vi "Obtain Control Cluster.vi"(9 "I/O":bool=TRUE, 10 "Dispense":bool=TRUE, 11 "Motion":bool=TRUE) -> (3 "Control Out":T1)   [LabVIEW 2020, in "Controller.lvclass"]
uses:
  Controller.lvclass
  Controllers.ctl
  I-O/I-O.lvclass
  Dispenser/Dispenser.lvclass
  C:/Program Files (x86)/Aerotech/A3200/LabVIEW/2010/Bin/Aerotech.A3200.dll
  Program Files (x86)/Aerotech/A3200/LabVIEW/2010/Bin/Aerotech.A3200.dll
  I-O/NI-DAQ/NI-DAQ.lvclass
  C:/Users/hep/Documents/CMU gantry/Classes/Controller/I-O/I-O.lvclass
  Dispenser/Ultimus V/Ultimus V.lvclass
  C:/Users/hep/Documents/CMU gantry/Classes/Controller/Dispenser/Dispenser.lvclass
panel:
  in  "Control":T1
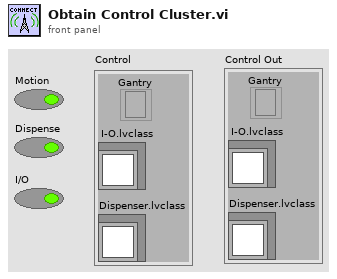
[diagram p1: front panel]
types:
  T1 = typedef "Controller.lvclass/Controllers.ctl" = cluster{"I-O.lvclass":refnum<class "I-O.lvclass">, "Dispenser.lvclass":refnum<class "Dispenser.lvclass">, "Gantry":refnum<k24>}
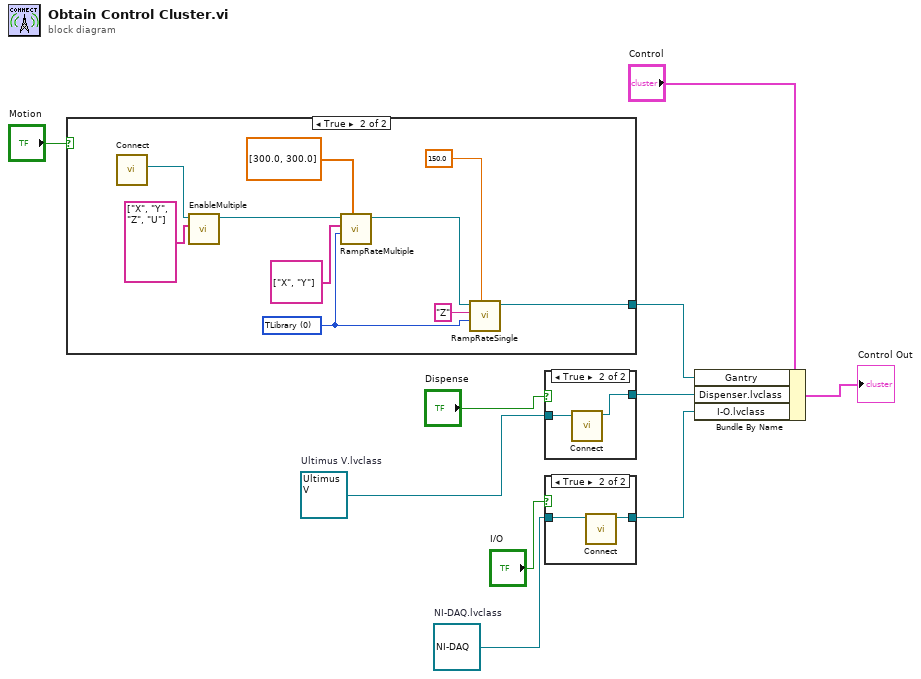
[diagram p0: block diagram]
diagram:
  w2 = refnum<class "Ultimus V.lvclass"> refnum  # Ultimus V.lvclass
  w5 = refnum<class "NI-DAQ.lvclass"> refnum  # NI-DAQ.lvclass
  n1 = case shown="True" "Motion" {
    tunnel: [_ w12] -> w3
    frame False {
    }
    frame True {
      w13 = 0 items=["TLibrary", "T01", "T02", "T03", "T04", "T05", "T06", "T07", "T08", "T09", "T10", "T11", "T12", "T13", "T14", "T15", "T16", "T17", "T18", "T19", "T20", "T21", "T22", "T23", "T24", "T25", "T26", "T27", "T28", "T29", "T30", "T31"] ("task id")
      n2 = call "Connect.vi"() -> ("controller"=w20:refnum<k24>)  [unwired: 10 in, 1 out]
      n3 = call "EnableMultiple.vi"("axis names"=string[] ["X", "Y", "Z", "U"], "controller in"=w20) -> ("controller out"=w18:refnum<k24>)  [unwired: 8 in, 1 out]
      n4 = call "RampRateMultiple.vi"("ramp rates"=dbl[] [300.0, 300.0], "task id"=w13, "axis names"=string[] ["X", "Y"], "controller in"=w18) -> ("controller out"=w15:refnum<k24>)  [unwired: 6 in, 1 out]
      n5 = call "RampRateSingle.vi"("ramp rate"=150.0, "task id"=w13, "axis name"="Z", "controller in"=w15) -> ("controller out"=w12:refnum<k24>)  [unwired: 6 in, 1 out]
    }
  }
  n6 = case shown="True" "Dispense" {
    tunnel: [w21 w22] -> w1
    tunnel: w2 -> [w21 w23]
    frame False {
    }
    frame True {
      n7 = call-dynamic "Connect.vi"("Ultimus V in"=w23) -> ("Ultimus V out"=w22:refnum<class "Ultimus V.lvclass">)  [unwired: 9 in, 1 out]
    }
  }
  n8 = case shown="True" "I/O" {
    tunnel: w5 -> [w24 w26]
    tunnel: [w24 w25] -> w8
    frame False {
    }
    frame True {
      n9 = call-dynamic "Connect.vi"("NI-DAQ in"=w26) -> ("NI-DAQ out"=w25:refnum<class "NI-DAQ.lvclass">)  [unwired: 9 in, 1 out]
    }
  }
  n10 = Bundle By Name(cluster="Control", "Gantry"=w3, "Dispenser.lvclass"=w1, "I-O.lvclass"=w8) -> (→"Control Out":T1)
